vi "ReadInstrumentsAddress.vi"(8 "error in (no error)":errorcluster, 11 "产品型号":refnum<vi>) -> (0 "error out":errorcluster, 4 "Instruments":T1(array[cluster]))   [LabVIEW 2013]
uses:
  SourceCode/GlobalValue.vi
  <vilib>/Utility/config.llb/Read Key (Boolean).vi
  <vilib>/Utility/config.llb/Read Key (String).vi
  <vilib>/Utility/config.llb/NI_LVConfig.lvlib
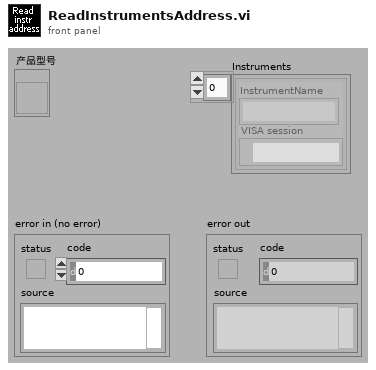
[diagram p1: front panel]
types:
  T1 = cluster{"InstrumentName":string, "VISA session":refnum<visa-resource-name>}[]
  T2 = typedef "NI_LVConfig.lvlib/Config Data RefNum.ctl" = refnum<k1>
  T3 = cluster{"InstrumentName":string, "VISA session":refnum<visa-resource-name>}
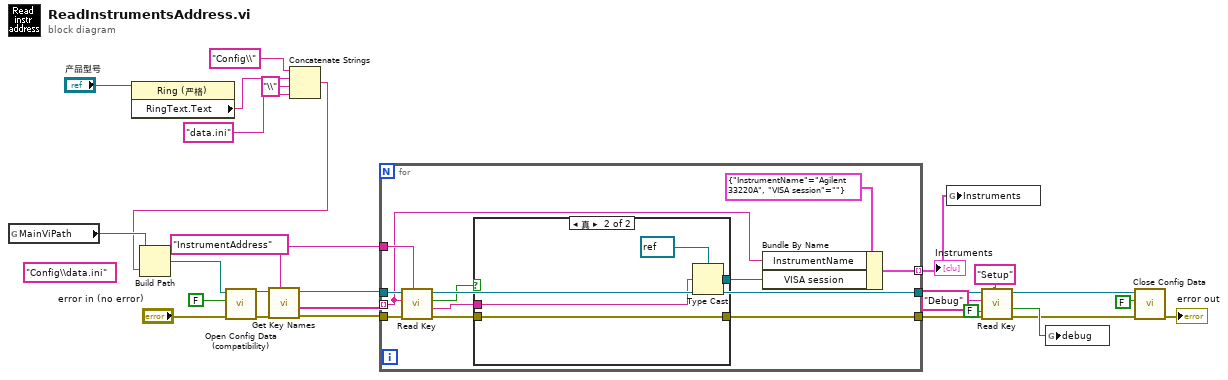
[diagram p0: block diagram]
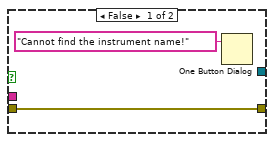
[diagram p2: hidden frame]
diagram:
  w18 = "InstrumentAddress" ("ModelName")
  (unwired) "Config\\data.ini" ("名称或相对路径")
  n1 = global read "GlobalValue.vi" "MainViPath"() -> (w15:path)
  n2 = property on="属性节点" class="Ring (严格)"(reference="产品型号") -> ("RingText.Text"=w11:string)  [unwired: 1 in, 2 out]
  n3 = Concatenate Strings("Config\\" ("名称或相对路径"), w11, "\\" ("字符串"), "data.ini" ("名称或相对路径")) -> (w9:string)
  n4 = Build Path(base path=w15, name or relative path=w9) -> (appended path=w24:path)
  n5 = call <vilib>:"Open Config Data (compatibility).vi"("error in (no error)"="error in (no error)", "create file if necessary (T)"=FALSE, "configuration file path"=w24) -> ("error out"=w22:errorcluster, "refnum"=w20:T2)  [unwired: 6 in, 1 out]
  n6 = call <vilib>:"Get Key Names.vi"("section"=w18, "error in (no error)"=w22, "refnum"=w20) -> ("error out"=w21:errorcluster, "key names"=w17:string[], "refnum out"=w19:T2)  [unwired: 5 in, 1 out]
  n7 = for {
    tunnel: w19 -> [w39]
    tunnel: w21 -> [w38]
    tunnel: [w37] -> w8
    tunnel: w17 -> [w30] mode=indexing
    tunnel: [w35] -> w7
    tunnel: w18 -> [w32]
    tunnel: [w28] -> w16 mode=indexing
    n8 = call-poly <vilib>:"Read Key.vi"("section"=w32, "error in (no error)"=w38, "key"=w30, "refnum"=w39) -> ("error out"=w34:errorcluster, "value"=w33:string, "found?"=w36:bool, "refnum out"=w37:T2)  [unwired: 2 in, 2 out]
    n9 = case shown="真" w36 {
      tunnel: [w40 w45] -> w35
      tunnel: w34 -> [w40 w45]
      tunnel: w33 -> [_ w44]
      tunnel: [_ w42] -> w29
      frame False {
        n10 = One Button Dialog(message="Cannot find the instrument name!" ("消息")) -> ()  [unwired: 2 out]
      }
      frame True {
        n11 = Type Cast(type=refnum<visa-resource-name> refnum ("VISA session"), x=w44) -> (*(type *) &x=w42:refnum<visa-resource-name>)
      }
    }
    n12 = Bundle By Name(cluster=T3 {"InstrumentName"="Agilent 33220A", "VISA session"=""}, "InstrumentName"=w30, "VISA session"=w29) -> (w28:T3)
  }
  "Instruments" <- w16
  n13 = global write "GlobalValue.vi" "Instruments"(w16) -> ()
  n14 = call-poly <vilib>:"Read Key.vi"("section"="Setup", "error in (no error)"=w7, "default value"=FALSE, "key"="Debug", "refnum"=w8) -> ("error out"=w1:errorcluster, "value"=w3:bool, "refnum out"=w2:T2)  [unwired: 4 out]
  n15 = global write "GlobalValue.vi" "debug"(w3) -> ()
  n16 = call <vilib>:"Close Config Data.vi"("error in (no error)"=w1, "write file if changed (T)"=FALSE ("write configuration file? (T)"), "refnum"=w2) -> ("error out"=→"error out":errorcluster)  [unwired: 8 out]
